vi "OPEN SERVO.vi"(4 "angle range":u16, 6 "servo PWM Channel":T2, 8 "error in (no error)":errorcluster, 9 "sub NT name":string, 10 "Zero angle":u16, 11 "servo refname":string) -> (0 "error out":errorcluster, 3 "ServoDeviceRef":T1={"DeviceStatus"={"status"=FALSE, "code"=0, "source"=""}, "PWM Channel"=enum."Invalid", "DeadBand"={"Name"="", "maxPositivePwm"=0, "minPositivePwm"=0, "centerPwm"=0, "maxNegativePwm"=0, "minNegativePwm"=0, "angularRange"=0}})   [LabVIEW 2020]
uses:
  <vilib>/Rock Robotics/Network Tables/NT Write Number.vi
  <vilib>/Rock Robotics/SystemInterfaces/DIO/FPGA_DIOPWMChannel.ctl
  <vilib>/Rock Robotics/WPI/PWM/WPI_PWMDeadband.ctl
  <vilib>/Rock Robotics/WPI/PWM/Servo/WPI_ServoDeviceRef.ctl
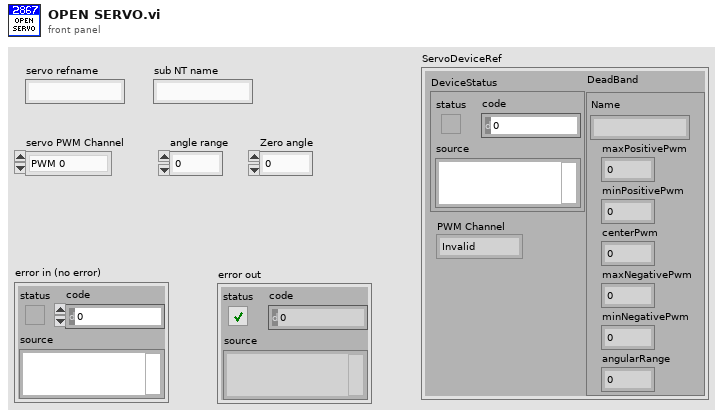
[diagram p1: front panel]
types:
  T1 = typedef "WPI_ServoDeviceRef.ctl" = cluster{"DeviceStatus":errorcluster, "PWM Channel":T2, "DeadBand":T3}
  T2 = typedef "FPGA_DIOPWMChannel.ctl" = enum8{"PWM 0", "PWM 1", "PWM 2", "PWM 3", "PWM 4", "PWM 5", "PWM 6", "PWM 7", "PWM 8", "PWM 9", "PWM MXP 0", "PWM MXP 1", "PWM MXP 2", "PWM MXP 3", "PWM MXP 4", "PWM MXP 5", "PWM MXP 6", "PWM MXP 7", "PWM MXP 8", "PWM MXP 9", "Invalid"}
  T3 = typedef "WPI_PWMDeadband.ctl" = cluster{"Name":string, "maxPositivePwm":i32, "minPositivePwm":i32, "centerPwm":i32, "maxNegativePwm":i32, "minNegativePwm":i32, "angularRange":u16}
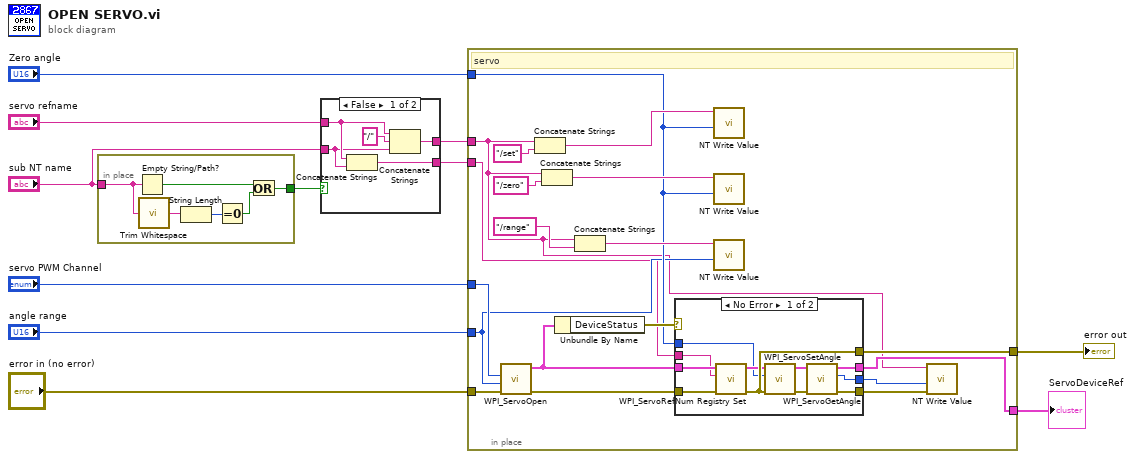
[diagram p0: block diagram]
diagram:
  n1 = in-place {
    in-place-border: [w13] -> w5
    in-place-border: "sub NT name" -> [w12]
    n2 = Empty String/Path?(string/path=w12) -> (empty?=w15:bool)
    n3 = call <vilib>:"Trim Whitespace.vi"("string"=w12) -> ("trimmed string"=w17:string)  [unwired: 1 in]
    n4 = String Length(string=w17) -> (length=w16:i32)
    n5 = Equal To 0?(x=w16) -> (x = 0?=w14:bool)
    n6 = Or(x=w15, y=w14) -> (x .or. y?=w13:bool)
  }
  n7 = case shown="False" w5 {
    tunnel: "servo refname" -> [w20 w23]
    tunnel: "sub NT name" -> [w19 _]
    tunnel: [w21 w23] -> w2
    tunnel: [w18 w23] -> w1
    frame False {
      n8 = Concatenate Strings(w20, w19) -> (w18:string)
      n9 = Concatenate Strings(w20, "/" ("string"), w19) -> (w21:string)
    }
    frame True {
    }
  }
  n10 = in-place {
    in-place-border: [w42] -> w8
    in-place-border: "Zero angle" -> [w30]
    in-place-border: "servo PWM Channel" -> [w29]
    in-place-border: "angle range" -> [w28]
    in-place-border: [w27] -> w7
    in-place-border: "error in (no error)" -> [w26]
    in-place-border: w2 -> [w25]
    in-place-border: w1 -> [w24]
    # "servo"
    n11 = call <vilib>:"WPI_ServoOpen.vi"("error in (no error)"=w26, "Angular Range"=w28, "PWM Channel"=w29) -> ("error out"=w33:errorcluster, "ServoDeviceRef"=w31:T1)  [unwired: 7 in]
    n12 = Concatenate Strings(w25, "/set" ("Name")) -> (w34:string)
    n13 = Concatenate Strings(w25, "/zero" ("string")) -> (w36:string)
    n14 = Unbundle By Name(w31) -> ("DeviceStatus"=w32:errorcluster)
    n15 = Concatenate Strings(w25, "/range" ("string")) -> (w37:string)
    n16 = case shown="No Error" w32 {
      tunnel: w31 -> [w53 _]
      tunnel: w24 -> [w52 _]
      tunnel: [w51 w54] -> w42
      tunnel: [w47 w54] -> w41
      tunnel: [w46 w55] -> w40
      tunnel: w30 -> [w45 w55]
      tunnel: w33 -> [w44 w54]
      tunnel: [w43 _] -> w27
      frame No Error {
        n17 = call <vilib>:"WPI_ServoRefNum Registry Set.vi"("error in (no error)"=w44, "refnum name"=w52, "ServoDeviceRef"=w53) -> ("error out"=w51:errorcluster, "ServoDeviceRef"=w50:T1)  [unwired: 7 in]
        n18 = call <vilib>:"WPI_ServoSetAngle.vi"("error in (no error)"=w51, "Angle"=w45, "ServoDeviceRef"=w50) -> ("error out"=w48:errorcluster, "ServoDeviceRef"=w49:T1)  [unwired: 7 in]
        n19 = call <vilib>:"WPI_ServoGetAngle.vi"("ServoDeviceRef"=w49, "error in (no error)"=w48) -> ("ServoDeviceRef"=w43:T1, "Angle"=w46:u16, "error out"=w47:errorcluster)  [unwired: 6 in]
      }
      frame Error {
      }
    }
    n20 = call-poly <vilib>:"NT Write Value.vi"("Numeric"=w30, "Name"=w34) -> ()  [unwired: 9 in, 1 out]
    n21 = call-poly <vilib>:"NT Write Value.vi"("Numeric"=w30, "Name"=w36) -> ()  [unwired: 9 in, 1 out]
    n22 = call-poly <vilib>:"NT Write Value.vi"("Numeric"=w28, "Name"=w37) -> ()  [unwired: 9 in, 1 out]
    n23 = call-poly <vilib>:"NT Write Value.vi"("error in"=w41, "Numeric"=w40, "Name"=w25) -> ()  [unwired: 8 in, 1 out]
  }
  "error out" <- w8
  "ServoDeviceRef" <- w7
